vi "demo.vi"() -> ()   [LabVIEW 2019]
uses:
  Fanfacade.ctl
panel:
  in  "Boolean":bool
  out "Fan":T1
  in  "stop":bool
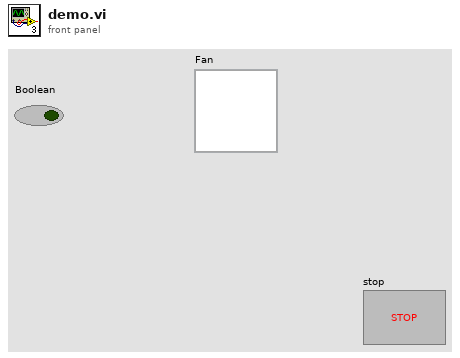
[diagram p1: front panel]
types:
  T1 = typedef "Fanfacade.ctl" = u16
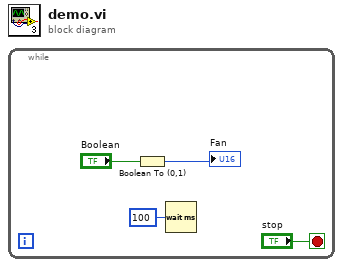
[diagram p0: block diagram]
diagram:
  n1 = while {
    stop <- "stop" stop-if-true
    n2 = Boolean To (0,1)(Boolean="Boolean") -> (0, 1=→"Fan":i16)
    n3 = Wait (ms)(milliseconds to wait=u32 100) -> ()  [unwired: 1 out]
  }
